vi "Measure Height_Mono Image Type.vi"(0 "Image In":T1, 3 "error in (no error)":errorcluster) -> (5 "Image":T1(plugin-control), 7 "Measurement on Right Spindle (Pixels)":dbl, 8 "Measurement on Centre Spindle (Pixels)":dbl, 9 "Measurement on Left Spindle (Pixels)":dbl, 10 "error out":errorcluster)   [LabVIEW 2016]
uses:
  <vilib>/vision/Image Controls.llb/IMAQ Image.ctl
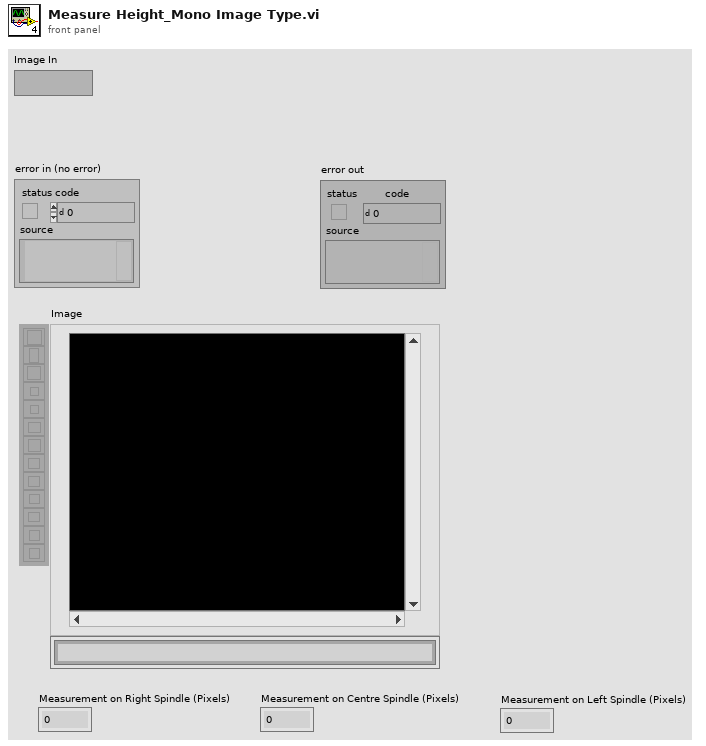
[diagram p1: front panel]
types:
  T1 = typedef "IMAQ Image.ctl" = refnum<image>
  T2 = cluster{"Distance (Pixels)":dbl, "Distance (Real World)":dbl, "Angle (Absolute)":dbl, "Angle (Relative)":dbl}
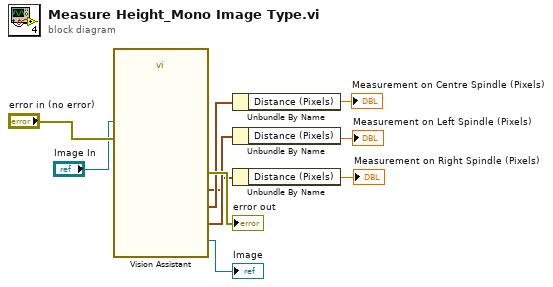
[diagram p0: block diagram]
diagram:
  n1 = call "Vision Assistant"("Image In"="Image In", "error in"="error in (no error)") -> ("Image Out"=→"Image":T1, "Clamp Results (Measurement of Right Spindle)"=w1:T2, "Clamp Results (Measurement of Center Spindle)"=w6:T2, "Clamp Results (Measurement of Left Spindle)"=w3:T2, "error out"=→"error out":errorcluster)  [unwired: 21 in]
  n2 = Unbundle By Name(w6) -> ("Distance (Pixels)"=→"Measurement on Centre Spindle (Pixels)":dbl)
  n3 = Unbundle By Name(w3) -> ("Distance (Pixels)"=→"Measurement on Left Spindle (Pixels)":dbl)
  n4 = Unbundle By Name(w1) -> ("Distance (Pixels)"=→"Measurement on Right Spindle (Pixels)":dbl)
